vi "QueueAction.vi"() -> ()   [LabVIEW 2011]
uses:
  UserEvent.ctl
  <userlib>/_OpenG.lib/numeric/numeric.llb/Random Number Within Range - DBL__ogtk.vi
panel:
  out "Numeric":u16
  in  "stop":bool
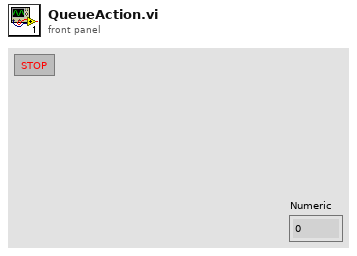
[diagram p1: front panel]
types:
  T1 = typedef "UserEvent.ctl" = cluster{"EventName":enum16{"USER_EVENT_1", "USER_EVENT_2", "USER_EVENT_3", "USER_EVENT_4", "USER_EVENT_5", "USER_EVENT_6", "USER_EVENT_7", "USER_EVENT_8", "USER_EVENT_9", "USER_EVENT_10"}, "Message":string, "EventData1":dbl, "EventData2":dbl}
  T2 = enum16{"USER_EVENT_1", "USER_EVENT_2", "USER_EVENT_3", "USER_EVENT_4", "USER_EVENT_5", "USER_EVENT_6", "USER_EVENT_7", "USER_EVENT_8", "USER_EVENT_9", "USER_EVENT_10"}
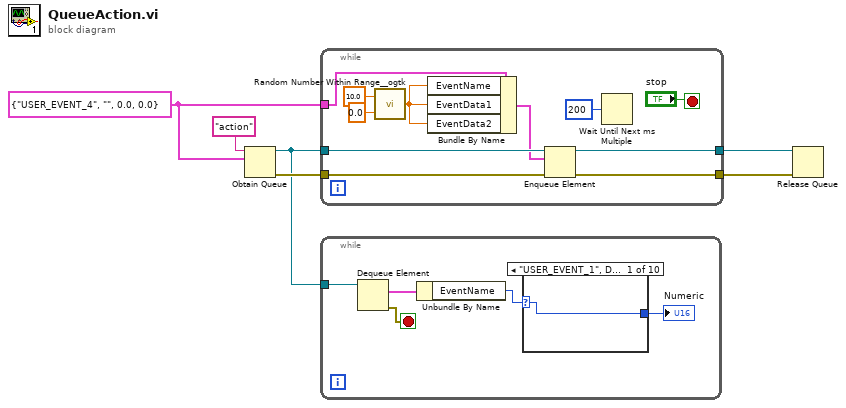
[diagram p0: block diagram]
diagram:
  w5 = T1 {"EventName"=enum."USER_EVENT_4", "Message"="", "EventData1"=0.0, "EventData2"=0.0} ("UserEvent")
  n1 = Obtain Queue(name (unnamed)="action", element data type=w5) -> (queue out=w1:refnum<queue>, error out=w4:errorcluster)  [unwired: 3 in, 1 out]
  n2 = while {
    tunnel: w1 -> [w16]
    tunnel: w5 -> [w14]
    tunnel: [w15] -> w3
    tunnel: w4 -> [w11]
    tunnel: [w10] -> w2
    stop <- "stop" stop-if-true
    n3 = call-poly <userlib>:"Random Number Within Range__ogtk.vi"("High"=10.0, "Low"=0.0) -> ("Random Number"=w13:dbl)  [unwired: 3 in]
    n4 = Bundle By Name(cluster=w14, "EventName"=w13, "EventData1"=w13, "EventData2"=w13) -> (w12:T1)
    n5 = Enqueue Element(queue=w16, element=w12, error in (no error)=w11) -> (queue out=w15:refnum<queue>, error out=w10:errorcluster)  [unwired: 1 in, 1 out]
    n6 = Wait Until Next ms Multiple(millisecond multiple=u32 200) -> ()  [unwired: 1 out]
  }
  n7 = while {
    tunnel: w1 -> [w22]
    stop <- w21 stop-if-true
    n8 = Dequeue Element(queue=w22) -> (element=w20:T1, error out=w21:errorcluster)  [unwired: 2 in, 2 out]
    n9 = Unbundle By Name(w20) -> ("EventName"=w19:T2)
    n10 = case shown="\"USER_EVENT_1\", Default" w19 {
      selector: w19 -> [w23 w24 w25 w26 w27 w28 w29 w30 w31 w32]
      tunnel: [w23 w24 w25 w26 w27 w28 w29 w30 w31 w32] -> w18
      frame "USER_EVENT_1", Default {
      }
      frame "USER_EVENT_2" {
      }
      frame "USER_EVENT_3" {
      }
      frame "USER_EVENT_4" {
      }
      frame "USER_EVENT_5" {
      }
      frame "USER_EVENT_6" {
      }
      frame "USER_EVENT_7" {
      }
      frame "USER_EVENT_8" {
      }
      frame "USER_EVENT_9" {
      }
      frame "USER_EVENT_10" {
      }
    }
    "Numeric" <- w18
  }
  n11 = Release Queue(queue=w3, error in (no error)=w2) -> ()  [unwired: 1 in, 3 out]
